vi "Remove Keyboard Filter.vi"(8 "error in (no error)":errorcluster) -> (0 "error out":errorcluster)   [LabVIEW 2023, in "WINKEY.lvlib"]
doc: "DOES NOT FUNCTION IN WIN32."
uses:
  WINKEY.lvlib
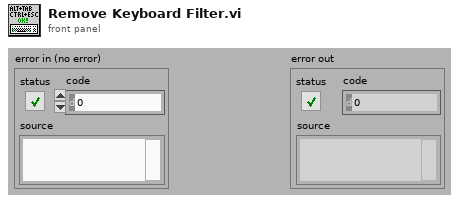
[diagram p1: front panel]
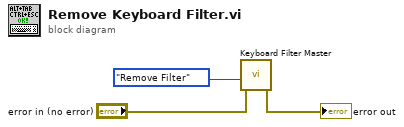
[diagram p0: block diagram]
diagram:
  n1 = call "Keyboard Filter Master.vi"("error in (no error)"="error in (no error)", "install / remove filter"=enum16{"Install Filter", "Remove Filter"}."Remove Filter") -> ("error out"=→"error out":errorcluster)  [unwired: 1 in, 2 out]
